vi "ziExample-ListDevices.vi"() -> ()   [LabVIEW 2009]
doc: "Control a Zurich instrument device via the LabOne Labview API. \nRequirements: Zurich Instruments MFLI, HF2 or UHFLI \nThis is an example for the Zurich Instruments LabOne LabVIEW API. This example lists all available instruments and displays some information on them.\n\n© Zurich Instruments AG, www.zhinst.com"
uses:
  <instrlib>/Zurich Instruments LabOne/Public/ziTypeDisovery.ctl
  <instrlib>/Zurich Instruments LabOne/Zurich Instruments LabOne.lvlib
panel:
  in  "Connect":bool
  out "Connected Device":string
  out "Error Out":errorcluster
  out "ziDiscovery":T1={"timestamp"=0, "deviceid"="", "devicetype"="", "serveraddress"="", "serverport"=0, "apilevel"=0, "discoverable"=TRUE, "interface"="", "connected"="", "available"=TRUE, "owner"="", "status"="", "options "="", "serverversion"=""}
  in  "stop":bool
  in  "Listbox":i32(listbox)
  # "ziExample-ListDevices.vi\nRequirements: HF2LI, UHFLI or MFLI\nsee block diagram for VI description"
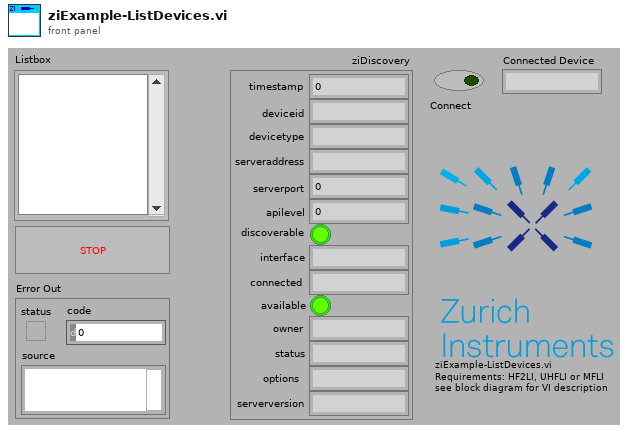
[diagram p1: front panel]
types:
  T1 = typedef "Zurich Instruments LabOne.lvlib/ziTypeDisovery.ctl" = cluster{"timestamp":u64, "deviceid":string, "devicetype":string, "serveraddress":string, "serverport":u32, "apilevel":u32, "discoverable":bool, "interface":string, "connected":string, "available":bool, "owner":string, "status":string, "options ":string, "serverversion":string}
  T2 = typedef "Zurich Instruments LabOne.lvlib/ziTypeHandle.ctl" = cluster{"handleValid":bool, "Conn":u64, "Path Prefix":string, "Handle":u64, "Connected":bool, "Clockbase(s)":dbl}
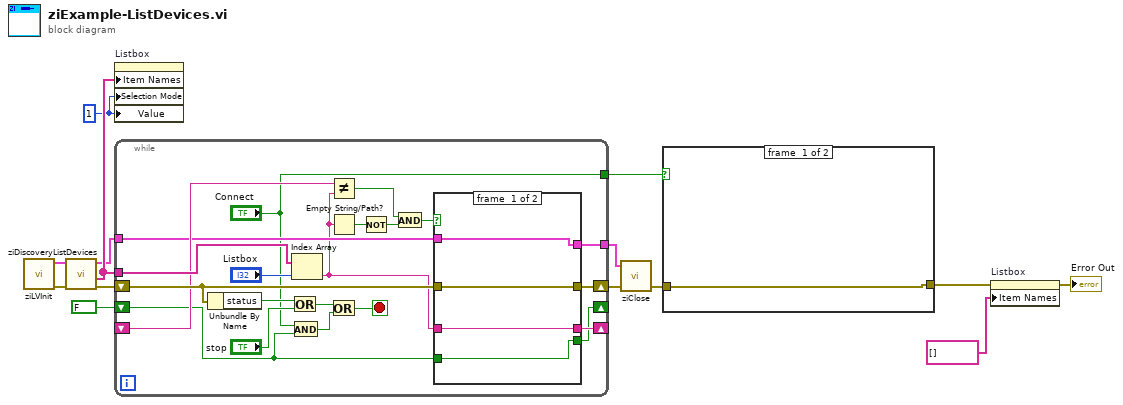
[diagram p0: block diagram]
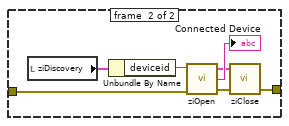
[diagram p2: hidden frame]
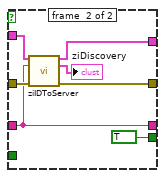
[diagram p3: hidden frame]
diagram:
  w10 = 1 ("Selection Mode")
  n1 = call <instrlib>:"ziLVInit.vi"() -> ("Error Out"=w14:errorcluster, "ziHandle"=w9:T2)  [unwired: 10 in]
  n2 = call <instrlib>:"ziDiscoveryListDevices.vi"("Error In"=w14, "ziHandle In"=w9) -> ("Error Out"=w12:errorcluster, "DevicesList"=w13:string[], "ziHandle Out"=w8:T2)  [unwired: 7 in]
  n3 = property on="Listbox" class="LstBox (strict)"("Item Names"=w13, "Selection Mode"=w10, "Value"=w10) -> ()  [unwired: 2 in, 2 out]
  n4 = while {
    tunnel: w13 -> [w34]
    shift-right: [w35] -> w11
    shift-left: w12 -> [w33]
    shift-right: [w30] -> _
    shift-left: _ -> [w29]
    tunnel: w8 -> [w26]
    tunnel: [w25] -> w7
    shift-right: [w23] -> _
    shift-left: FALSE -> [w22]
    tunnel: ["Connect"] -> w5
    stop <- w20 stop-if-true
    n5 = Unbundle By Name(w33) -> ("status"=w32:bool)
    n6 = Or(x=w32, y="stop") -> (x .or. y?=w21:bool)
    n7 = And(x="Connect", y=w22) -> (x .and. y?=w19:bool)
    n8 = Index Array(array=w34, index="Listbox") -> (element=w16:string)
    n9 = Not Equal?(x=w29, y=w16) -> (x != y?=w28:bool)
    n10 = Empty String/Path?(string/path=w16) -> (empty?=w17:bool)
    n11 = Or(x=w21, y=w19) -> (x .or. y?=w20:bool)
    n12 = Not(x=w17) -> (.not. x?=w15:bool)
    n13 = And(x=w28, y=w15) -> (x .and. y?=w27:bool)
    n14 = case shown="True" w27 {
      tunnel: [w38 w46] -> w35
      tunnel: w16 -> [w39 w43]
      tunnel: w33 -> [w38 w45]
      tunnel: [w39 w43] -> w30
      tunnel: w26 -> [w37 w42]
      tunnel: [w37 w41] -> w25
      tunnel: w22 -> [w36 _]
      tunnel: [w36 TRUE] -> w23
      frame #0 {
      }
      frame #1 {
        n15 = call <instrlib>:"ziIDToServer.vi"("ziHandle In"=w42, "Device ID"=w43, "Error In"=w45) -> ("ziHandle Out"=w41:T2, "ziDiscovery"=→"ziDiscovery":T1, "Error Out"=w46:errorcluster)  [unwired: 10 in]
      }
    }
  }
  n16 = call <instrlib>:"ziClose.vi"("Error In"=w11, "Handle In"=w7) -> ("Error Out"=w4:errorcluster)  [unwired: 2 in, 1 out]
  n17 = case shown="True" w5 {
    tunnel: [w47 w50] -> w2
    tunnel: w4 -> [w47 w49]
    frame #0 {
    }
    frame #1 {
      n18 = local read "ziDiscovery"() -> (w51:T1)
      n19 = Unbundle By Name(w51) -> ("deviceid"=w48:string)
      n20 = call <instrlib>:"ziOpen.vi"("Error In"=w49, "Address"=w48) -> ("Error Out"=w52:errorcluster, "Selected Device"=→"Connected Device":string, "HandleOut"=w53:T2)  [unwired: 2 in]
      n21 = call <instrlib>:"ziClose.vi"("Error In"=w52, "Handle In"=w53) -> ("Error Out"=w50:errorcluster)  [unwired: 2 in, 1 out]
    }
  }
  n22 = property on="Listbox" class="LstBox (strict)"(error in=w2, "Item Names"=string[] []) -> (error out=→"Error Out":errorcluster)  [unwired: 1 in, 1 out]
